vi "Notify to MS teams.vi"(9 "message":string, 10 "title":string, 11 "URL":string) -> ()   [LabVIEW 2022 SP3]
uses:
  <vilib>/httpClient/POSTBuffer.vi
  <vilib>/httpClient/LabVIEWHTTPClient.lvlib
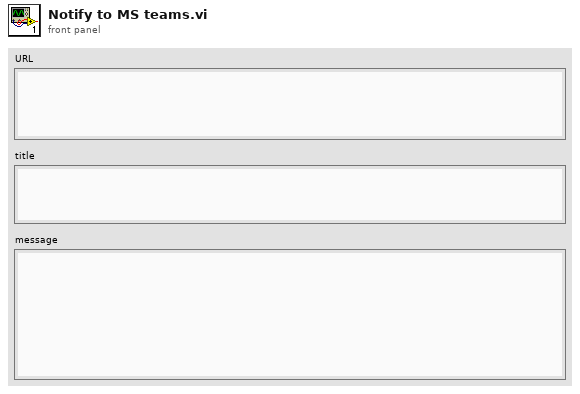
[diagram p1: front panel]
types:
  T1 = cluster{"attachments":cluster{"contentType":string, "content":cluster{"$schema":string, "type":string, "version":string, "body":cluster{"type":string, "size":string, "weight":string, "text":string, "wrap":bool, "markdown":bool}[]}}[]}
  T2 = cluster{"contentType":string, "content":cluster{"$schema":string, "type":string, "version":string, "body":cluster{"type":string, "size":string, "weight":string, "text":string, "wrap":bool, "markdown":bool}[]}}[]
  T3 = cluster{"contentType":string, "content":cluster{"$schema":string, "type":string, "version":string, "body":cluster{"type":string, "size":string, "weight":string, "text":string, "wrap":bool, "markdown":bool}[]}}
  T4 = cluster{"type":string, "size":string, "weight":string, "text":string, "wrap":bool, "markdown":bool}[]
  T5 = cluster{"type":string, "size":string, "weight":string, "text":string, "wrap":bool, "markdown":bool}
  T6 = typedef "LabVIEWHTTPClient.lvlib/ClientHandle.ctl" = refnum<k1>
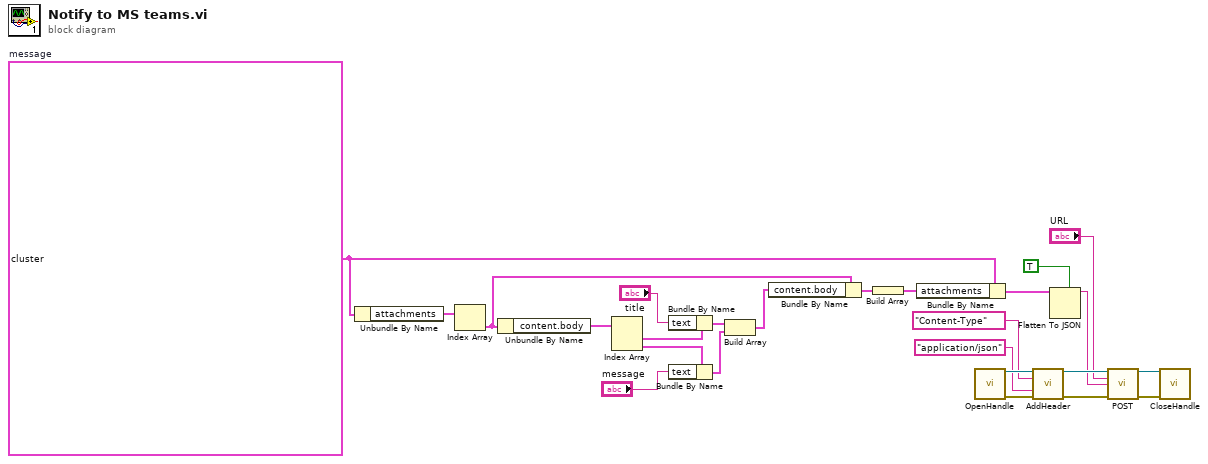
[diagram p0: block diagram]
diagram:
  w3 = T1 {"attachments"=[{"contentType"="application/vnd.microsoft.card.adaptive", "content"={"$schema"="http://adaptivecards.io/schemas/adaptive-card.json", "type"="AdaptiveCard", "version"="1.2", "body"=[{"type"="TextBlock", "size"="Medium", "weight"="Bolder", "text"="", "wrap"=TRUE, "markdown"=TRUE}, {"type"="TextBlock", "size"="", "weight"="", "text"="", "wrap"=TRUE, "markdown"=TRUE}]}}]}  # message
  n1 = Unbundle By Name(w3) -> ("attachments"=w14:T2)
  n2 = Index Array(array=w14) -> (element=w6:T3)  [unwired: 1 in]
  n3 = Unbundle By Name(w6) -> ("content.body"=w13:T4)
  n4 = Index Array(array=w13) -> (element #1=w12:T5, element #2=w10:T5)  [unwired: 2 in]
  n5 = Bundle By Name(cluster=w12, "text"="title") -> (w8:T5)
  n6 = Bundle By Name(cluster=w10, "text"="message") -> (w7:T5)
  n7 = Build Array(w8, w7) -> (w5:T4)
  n8 = Bundle By Name(cluster=w6, "content.body"=w5) -> (w4:T3)
  n9 = Build Array(w4) -> (w2:T2)
  n10 = Bundle By Name(cluster=w3, "attachments"=w2) -> (w1:T1)
  n11 = call <vilib>:"OpenHandle.vi"() -> ("client handle out"=w25:T6, "error out"=w24:errorcluster)  [unwired: 14 in]
  n12 = call <vilib>:"AddHeader.vi"("client handle"=w25, "header"="Content-Type", "value"="application/json", "error in (no error)"=w24) -> ("client handle out"=w22:T6, "error out"=w23:errorcluster)  [unwired: 10 in]
  n13 = Flatten To JSON(enable LabVIEW extensions? (T)=TRUE, anything=w1) -> (JSON string=w17:string)  [unwired: 1 in, 1 out]
  n14 = call-poly <vilib>:"POST.vi"("client handle"=w22, "url"="URL", "buffer"=w17, "error in (no error)"=w23) -> ("client handle out"=w21:T6, "error out"=w20:errorcluster)  [unwired: 8 in, 2 out]
  n15 = call <vilib>:"CloseHandle.vi"("client handle"=w21, "error in (no error)"=w20) -> ()  [unwired: 13 in, 1 out]
